vi "Array of Scalar.vi"(6 "Type":T1, 8 "error in (no error)":errorcluster, 9 "Array Element Data Type":variant, 10 "Element Offsets":i32[](array[numeric]), 11 "JSON":string) -> (0 "error out":errorcluster, 3 "Array":variant[](array[variant]))   [LabVIEW 2024, in "JSONtext.lvlib"]
uses:
  JSONtext.lvlib
  Data Type.ctl
  Get String.vi
  Get DBL.vi
  Get Timestamp.vi
  Get I8.vi
  Get I16.vi
  Get I32.vi
  Get I64.vi
  Get U8.vi
  Get U16.vi
  Get U32.vi
  Get U64.vi
  Get Boolean.vi
  Coerce I32 to Variant Intger.vi
  Format Error.vi
  Get SGL.vi
  Advance past String.vi
  String Subset.vi
  Strip Quotes and Unescape.vi
  Get Number Text.vi
  Advance past whitespace.vi
  NaN or null to Integer ERROR.vi
  Advance past Number.vi
  Unescape JSON string.vi
  Advance past Line Ending.vi
  Error Cluster From Error Code.vi
  Parsing Error in converting to LabVIEW type.vi
  JSON type.vi
  Get Refnum Information.vi
  Error Cluster From Code.vi
  Text to Timestamp.vi
  Get Numeric Information.vi
  Get Type Information.vi
  NI_Data Type.lvlib
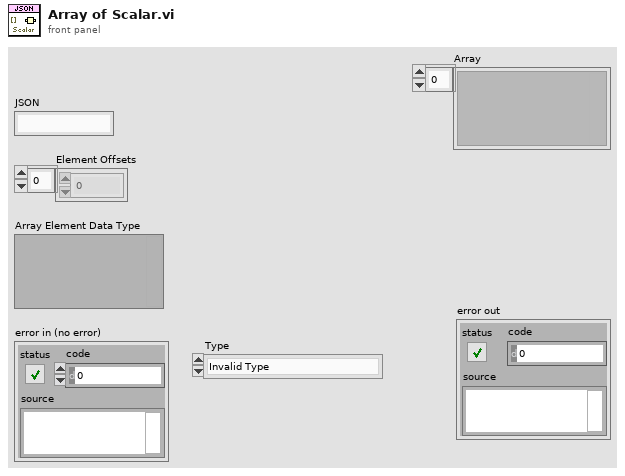
[diagram p1: front panel]
types:
  T1 = typedef "NI_Data Type.lvlib/Data Type.ctl" = enum8{"Invalid Type", "Void", "I8", "I16", "I32", "I64", "U8", "U16", "U32", "U64", "Single Float", "Double Float", "Extended Float", "Single Complex", "Double Complex", "Extended Complex", "Enum U8", "Enum U16", "Enum U32", "Enum U64", "Single Float With Unit", "Double Float With Unit", "Extended Float With Unit", "Single Complex with Unit", "Double Complex with Unit", "Extended Complex with Unit", "Boolean", "String", "Path", "Picture", "Tag", "Array", "Cluster", "Variant", "LV Variant", "Waveform", "Timestamp", "Digital Waveform", "Digital Data", "ExpressData", "Refnum", "External Data", "VI", "Poly VI", "LabVIEW Class Instance", "Fixed Point", "Set Collection", "Map Collection"}
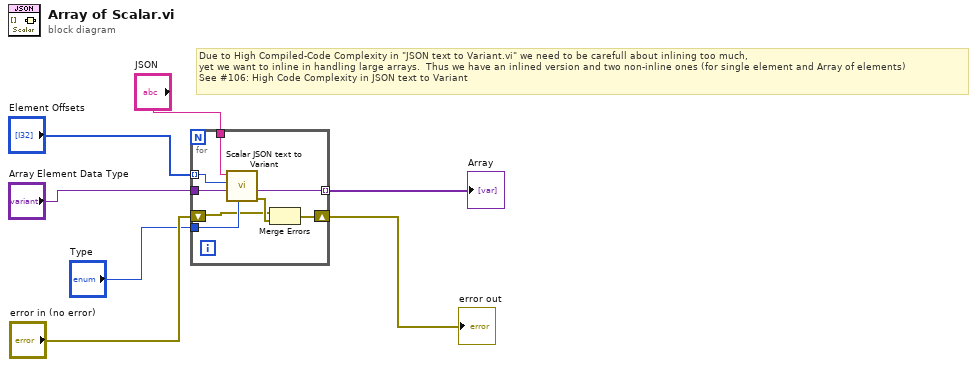
[diagram p0: block diagram]
diagram:
  # "Due to High Compiled-Code Complexity in \"JSON text to Variant.vi\" we need to be carefull about inlining too much,\nyet we want to inline in handling large arrays.  Thus we have an inlined version and two non-inline ones (for single element and Array of elements)\nSee #106: High Code Complexity in JSON text to Variant"
  n1 = for {
    tunnel: "Array Element Data Type" -> [w15]
    tunnel: [w14] -> w4 mode=indexing
    tunnel: "Element Offsets" -> [w11] mode=indexing
    tunnel: "Type" -> [w12]
    tunnel: "JSON" -> [w10]
    shift-right: [w9] -> w1
    shift-left: "error in (no error)" -> [w8]
    n2 = call "Scalar JSON text to Variant.vi"("Type"=w12, "Variant (Data Type)"=w15, "Offset (no whitespace)"=w11, "JSON"=w10) -> ("error out"=w13:errorcluster, "Variant out"=w14:variant)  [unwired: 6 in]
    n3 = Merge Errors(w8, w13) -> (w9:errorcluster)
  }
  "Array" <- w4
  "error out" <- w1
